vi "Launch.vi"(8 "error in":errorcluster, 11 "Philips Dialog in":refnum<class "Flex UI Dialog.lvclass">) -> (0 "error out":errorcluster, 3 "Philips Dialog out":refnum<class "Flex UI Dialog.lvclass">)   [LabVIEW 2014, in "Flex UI Dialog.lvclass"]
doc: "Launches the UI."
uses:
  Flex UI Dialog.lvclass
  Flex UI Dialog.lvclass/Flex UI Dialog.ctl
  Flex UI (Parent)/Flex UI.lvclass
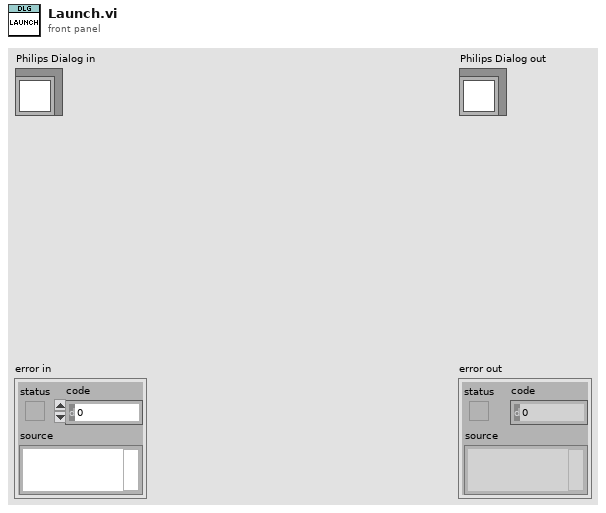
[diagram p1: front panel]
types:
  T1 = typedef "Flex UI Dialog.lvclass/Enum - Launch Position.ctl" = enum16{"Default (Last Opened)", "Centered", "Centered on Caller", "Maximized", "Hidden"}
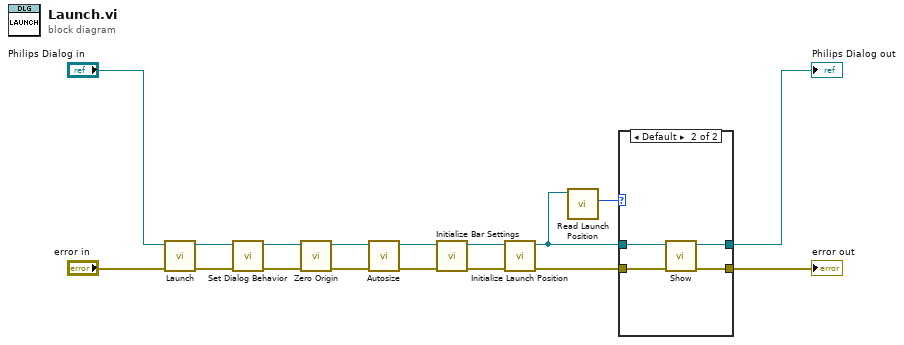
[diagram p0: block diagram]
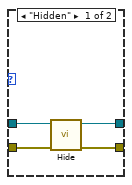
[diagram p2: hidden frame]
diagram:
  n1 = call-parent "Launch.vi"("error in"="error in", "Philips UI in"="Philips Dialog in") -> ("error out"=w8:errorcluster, "Philips UI out"=w5:refnum<class "Flex UI Dialog.lvclass">)  [unwired: 8 in]
  n2 = call "Set Dialog Behavior.vi"("error in"=w8, "Philips Dialog in"=w5) -> ("error out"=w17:errorcluster, "Philips Dialog out"=w12:refnum<class "Flex UI Dialog.lvclass">)  [unwired: 8 in]
  n3 = call "Zero Origin.vi"("error in"=w17, "Philips UI in"=w12) -> ("error out"=w13:errorcluster, "Philips UI out"=w11:refnum<class "Flex UI Dialog.lvclass">)  [unwired: 8 in]
  n4 = call-dynamic "Autosize.vi"("error in"=w13, "Philips Dialog in"=w11) -> ("error out"=w14:errorcluster, "Philips Dialog out"=w9:refnum<class "Flex UI Dialog.lvclass">)  [unwired: 8 in]
  n5 = call "Initialize Bar Settings.vi"("error in"=w14, "Philips Dialog in"=w9) -> ("error out"=w10:errorcluster, "Philips Dialog out"=w3:refnum<class "Flex UI Dialog.lvclass">)  [unwired: 8 in]
  n6 = call-dynamic "Initialize Launch Position.vi"("error in"=w10, "Philips Dialog in"=w3) -> ("error out"=w4:errorcluster, "Philips Dialog out"=w2:refnum<class "Flex UI Dialog.lvclass">)  [unwired: 8 in]
  n7 = call "Read Launch Position.vi"("Philips Dialog in"=w2) -> ("Launch Position"=w1:T1)  [unwired: 9 in, 1 out]
  n8 = case shown="Default" w1 {
    tunnel: [w20 w25] -> w16
    tunnel: [w18 w24] -> w15
    tunnel: w4 -> [w21 w23]
    tunnel: w2 -> [w19 w22]
    frame "Hidden" {
      n9 = call-dynamic "Hide.vi"("error in"=w21, "Philips Dialog in"=w19) -> ("error out"=w20:errorcluster, "Philips Dialog out"=w18:refnum<class "Flex UI Dialog.lvclass">)  [unwired: 8 in]
    }
    frame Default {
      n10 = call-dynamic "Show.vi"("error in"=w23, "Philips Dialog in"=w22) -> ("error out"=w25:errorcluster, "Philips Dialog out"=w24:refnum<class "Flex UI Dialog.lvclass">)  [unwired: 8 in]
    }
  }
  "error out" <- w16
  "Philips Dialog out" <- w15
